vi "gxml_BlindXMLtoFlatString.vi"(6 "Encaps Array Info":T1, 8 "error in":errorcluster, 9 "Item Name":cluster{"Hierarchy":string, "Item Name":string}, 10 "Datatype":string, 11 "Item Contents":string) -> (0 "error out":errorcluster, 2 "XML Data (Flat Str)":string)   [LabVIEW 2011, in "Third Party VIs.lvlib" / "GXML.lvlib"]
uses:
  GXML.lvlib
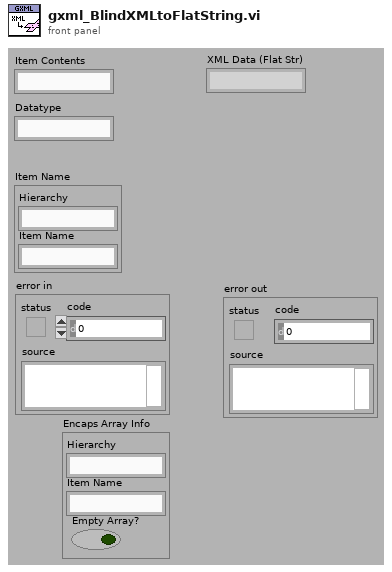
[diagram p1: front panel]
types:
  T1 = cluster{"Hierarchy":string, "Item Name":string, "Empty Array?":bool}
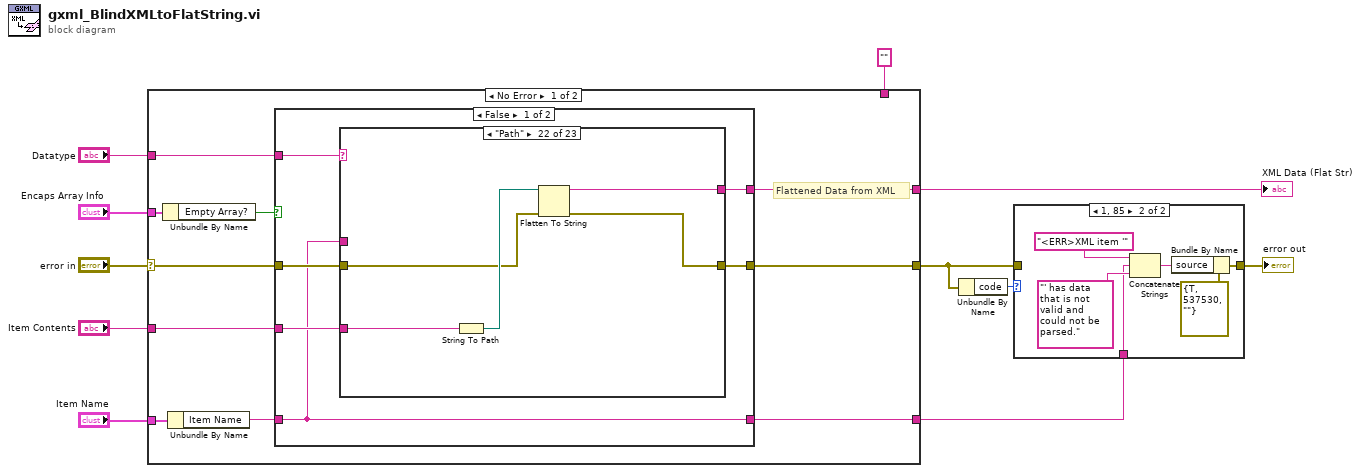
[diagram p0: block diagram]
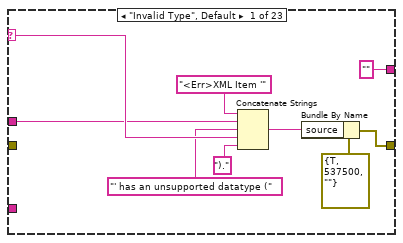
[diagram p3: hidden frame]
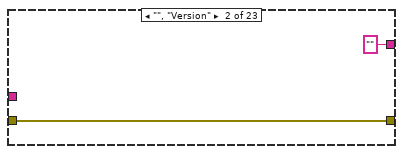
[diagram p4: hidden frame]
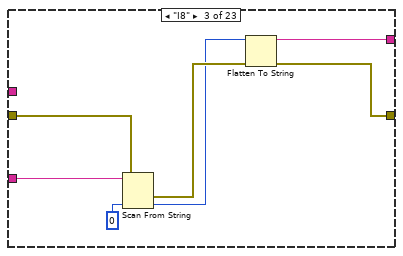
[diagram p5: hidden frame]
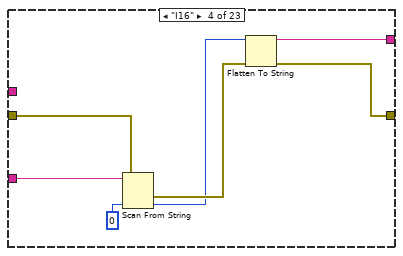
[diagram p6: hidden frame]
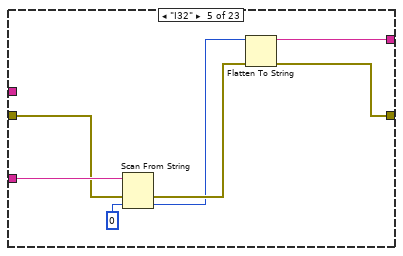
[diagram p7: hidden frame]
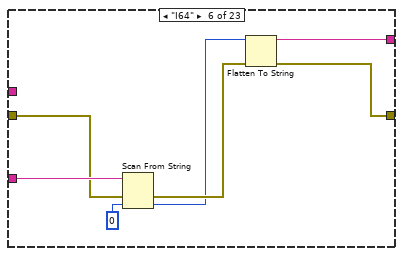
[diagram p8: hidden frame]
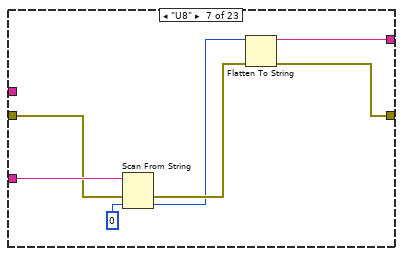
[diagram p9: hidden frame]
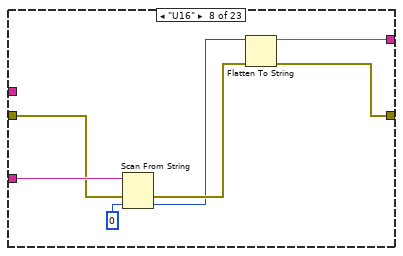
[diagram p10: hidden frame]
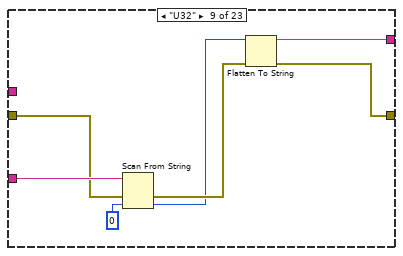
[diagram p11: hidden frame]
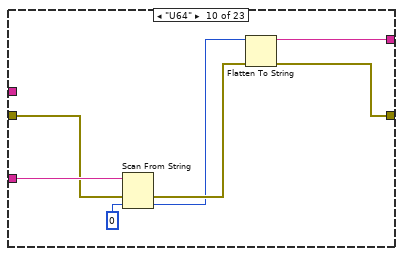
[diagram p12: hidden frame]
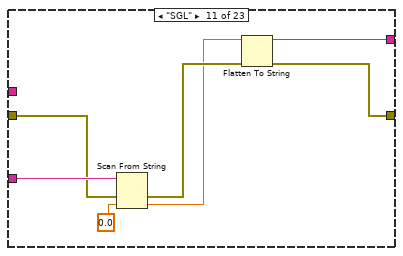
[diagram p13: hidden frame]
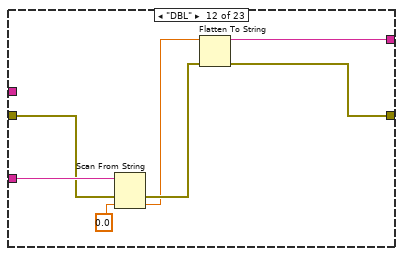
[diagram p14: hidden frame]
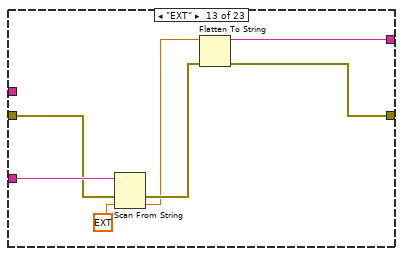
[diagram p15: hidden frame]
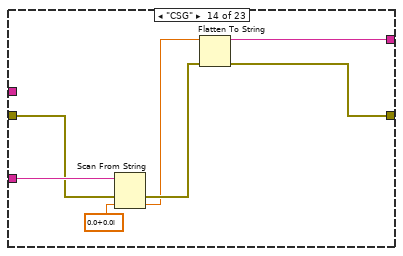
[diagram p16: hidden frame]
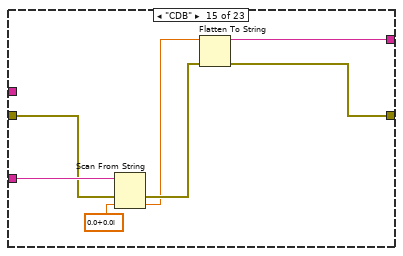
[diagram p17: hidden frame]
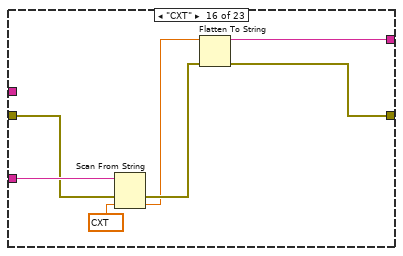
[diagram p18: hidden frame]
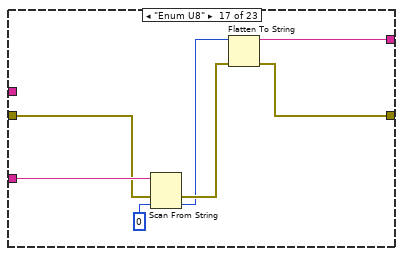
[diagram p19: hidden frame]
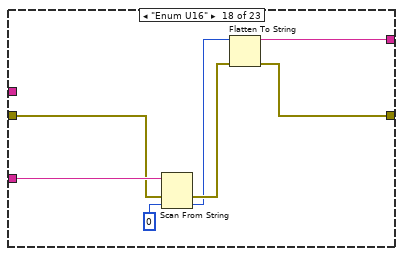
[diagram p20: hidden frame]
diagram:
  n1 = case shown="No Error" "error in" {
    selector: "error in" -> [w17 w191]
    tunnel: [w20 w191] -> w5
    tunnel: [w21 w190] -> w11
    tunnel: "Datatype" -> [w18 _]
    tunnel: "Item Contents" -> [w19 _]
    tunnel: "" ("data string") -> [_ w190]
    tunnel: "Item Name" -> [w16 _]
    tunnel: [w13 w190] -> w2
    tunnel: "Encaps Array Info" -> [w14 _]
    frame No Error {
      # "Flattened Data from XML"
      n2 = Unbundle By Name(w14) -> ("Empty Array?"=w12:bool)
      n3 = Unbundle By Name(w16) -> ("Item Name"=w15:string)
      n4 = case shown="False" w12 {
        tunnel: [w27 "" ("data string")] -> w21
        tunnel: [w26 w188] -> w20
        tunnel: w19 -> [w25 _]
        tunnel: w18 -> [w24 _]
        tunnel: w17 -> [w23 w188]
        tunnel: w15 -> [w22 w189]
        tunnel: [w22 w189] -> w13
        frame False {
          n5 = case shown="\"Path\"" w24 {
            selector: w24 -> [w33 _ _ _ _ _ _ _ _ _ _ _ _ _ _ _ _ _ _ _ _ _ _]
            tunnel: ["" ("data string") "" ("data string") w42 w49 w56 w63 w70 w77 w84 w91 w100 w107 w114 w121 w128 w135 w140 w147 w154 w163 w168 w173 w185] -> w27
            tunnel: [w34 w38 w41 w48 w55 w62 w69 w76 w83 w90 w101 w108 w115 w122 w129 w136 w137 w144 w152 w164 w169 w174 w186] -> w26
            tunnel: w25 -> [_ _ w44 w51 w58 w65 w72 w79 w86 w93 w98 w105 w112 w119 w126 w133 w143 w150 w157 w162 w165 w172 w178]
            tunnel: w23 -> [_ w38 w43 w50 w57 w64 w71 w78 w85 w92 w95 w102 w109 w116 w123 w130 w138 w145 w151 w158 w167 w170 w179]
            tunnel: w22 -> [w28 _ _ _ _ _ _ _ _ _ _ _ _ _ _ _ _ _ _ _ _ _ w177]
            frame "Invalid Type", Default {
              n6 = Concatenate Strings("<Err>XML Item '", w28, "' has an unsupported datatype (" ("string"), w33, ")." ("string")) -> (w32:string)
              n7 = Bundle By Name(cluster=errorcluster {"status"=TRUE, "code"=537500, "source"=""} ("error out"), "source"=w32) -> (w34:errorcluster)
            }
            frame "", "Version" {
            }
            frame "I8" {
              n8 = Scan From String(input string=w44, error in=w43, default 1=i8 0) -> (error out=w40:errorcluster, output 1=w39:i8)  [unwired: 2 in, 2 out]
              n9 = Flatten To String(anything=w39, error in (no error)=w40) -> (data string=w42:string, error out=w41:errorcluster)  [unwired: 2 in, 1 out]
            }
            frame "I16" {
              n10 = Scan From String(input string=w51, error in=w50, default 1=i16 0) -> (error out=w47:errorcluster, output 1=w46:i16)  [unwired: 2 in, 2 out]
              n11 = Flatten To String(anything=w46, error in (no error)=w47) -> (data string=w49:string, error out=w48:errorcluster)  [unwired: 2 in, 1 out]
            }
            frame "I32" {
              n12 = Scan From String(input string=w58, error in=w57, default 1=0) -> (error out=w54:errorcluster, output 1=w53:i32)  [unwired: 2 in, 2 out]
              n13 = Flatten To String(anything=w53, error in (no error)=w54) -> (data string=w56:string, error out=w55:errorcluster)  [unwired: 2 in, 1 out]
            }
            frame "I64" {
              n14 = Scan From String(input string=w65, error in=w64, default 1=i64 0) -> (error out=w61:errorcluster, output 1=w60:i64)  [unwired: 2 in, 2 out]
              n15 = Flatten To String(anything=w60, error in (no error)=w61) -> (data string=w63:string, error out=w62:errorcluster)  [unwired: 2 in, 1 out]
            }
            frame "U8" {
              n16 = Scan From String(input string=w72, error in=w71, default 1=u8 0) -> (error out=w68:errorcluster, output 1=w67:u8)  [unwired: 2 in, 2 out]
              n17 = Flatten To String(anything=w67, error in (no error)=w68) -> (data string=w70:string, error out=w69:errorcluster)  [unwired: 2 in, 1 out]
            }
            frame "U16" {
              n18 = Scan From String(input string=w79, error in=w78, default 1=u16 0) -> (error out=w75:errorcluster, output 1=w74:u16)  [unwired: 2 in, 2 out]
              n19 = Flatten To String(anything=w74, error in (no error)=w75) -> (data string=w77:string, error out=w76:errorcluster)  [unwired: 2 in, 1 out]
            }
            frame "U32" {
              n20 = Scan From String(input string=w86, error in=w85, default 1=u32 0) -> (error out=w82:errorcluster, output 1=w81:u32)  [unwired: 2 in, 2 out]
              n21 = Flatten To String(anything=w81, error in (no error)=w82) -> (data string=w84:string, error out=w83:errorcluster)  [unwired: 2 in, 1 out]
            }
            frame "U64" {
              n22 = Scan From String(input string=w93, error in=w92, default 1=u64 0) -> (error out=w89:errorcluster, output 1=w88:u64)  [unwired: 2 in, 2 out]
              n23 = Flatten To String(anything=w88, error in (no error)=w89) -> (data string=w91:string, error out=w90:errorcluster)  [unwired: 2 in, 1 out]
            }
            frame "SGL" {
              n24 = Scan From String(input string=w98, error in=w95, default 1=sgl 0.0) -> (error out=w97:errorcluster, output 1=w96:sgl)  [unwired: 2 in, 2 out]
              n25 = Flatten To String(anything=w96, error in (no error)=w97) -> (data string=w100:string, error out=w101:errorcluster)  [unwired: 2 in, 1 out]
            }
            frame "DBL" {
              n26 = Scan From String(input string=w105, error in=w102, default 1=0.0) -> (error out=w104:errorcluster, output 1=w103:dbl)  [unwired: 2 in, 2 out]
              n27 = Flatten To String(anything=w103, error in (no error)=w104) -> (data string=w107:string, error out=w108:errorcluster)  [unwired: 2 in, 1 out]
            }
            frame "EXT" {
              n28 = Scan From String(input string=w112, error in=w109, default 1=ext 0.0) -> (error out=w111:errorcluster, output 1=w110:ext)  [unwired: 2 in, 2 out]
              n29 = Flatten To String(anything=w110, error in (no error)=w111) -> (data string=w114:string, error out=w115:errorcluster)  [unwired: 2 in, 1 out]
            }
            frame "CSG" {
              n30 = Scan From String(input string=w119, error in=w116, default 1=csg 0.0+0.0i) -> (error out=w118:errorcluster, output 1=w117:csg)  [unwired: 2 in, 2 out]
              n31 = Flatten To String(anything=w117, error in (no error)=w118) -> (data string=w121:string, error out=w122:errorcluster)  [unwired: 2 in, 1 out]
            }
            frame "CDB" {
              n32 = Scan From String(input string=w126, error in=w123, default 1=cdb 0.0+0.0i) -> (error out=w125:errorcluster, output 1=w124:cdb)  [unwired: 2 in, 2 out]
              n33 = Flatten To String(anything=w124, error in (no error)=w125) -> (data string=w128:string, error out=w129:errorcluster)  [unwired: 2 in, 1 out]
            }
            frame "CXT" {
              n34 = Scan From String(input string=w133, error in=w130, default 1=cxt 0.0+0.0i) -> (error out=w132:errorcluster, output 1=w131:cxt)  [unwired: 2 in, 2 out]
              n35 = Flatten To String(anything=w131, error in (no error)=w132) -> (data string=w135:string, error out=w136:errorcluster)  [unwired: 2 in, 1 out]
            }
            frame "Enum U8" {
              n36 = Scan From String(input string=w143, error in=w138, default 1=u8 0) -> (error out=w141:errorcluster, output 1=w139:u8)  [unwired: 2 in, 2 out]
              n37 = Flatten To String(anything=w139, error in (no error)=w141) -> (data string=w140:string, error out=w137:errorcluster)  [unwired: 2 in, 1 out]
            }
            frame "Enum U16" {
              n38 = Scan From String(input string=w150, error in=w145, default 1=u16 0) -> (error out=w148:errorcluster, output 1=w146:u16)  [unwired: 2 in, 2 out]
              n39 = Flatten To String(anything=w146, error in (no error)=w148) -> (data string=w147:string, error out=w144:errorcluster)  [unwired: 2 in, 1 out]
            }
            frame "Enum U32" {
              n40 = Scan From String(input string=w157, error in=w151, default 1=u32 0) -> (error out=w155:errorcluster, output 1=w153:u32)  [unwired: 2 in, 2 out]
              n41 = Flatten To String(anything=w153, error in (no error)=w155) -> (data string=w154:string, error out=w152:errorcluster)  [unwired: 2 in, 1 out]
            }
            frame "Bool" {
              n42 = Scan From String(input string=w162, error in=w158, default 1=FALSE) -> (error out=w160:errorcluster, output 1=w159:bool)  [unwired: 2 in, 2 out]
              n43 = Flatten To String(anything=w159, error in (no error)=w160) -> (data string=w163:string, error out=w164:errorcluster)  [unwired: 2 in, 1 out]
            }
            frame "String", "Tag" {
              n44 = call "gxml_UnescapeChar.vi"("XML In"=w165) -> ("XML Out"=w166:string)  [unwired: 10 in]
              n45 = Flatten To String(anything=w166, error in (no error)=w167) -> (data string=w168:string, error out=w169:errorcluster)  [unwired: 2 in, 1 out]
            }
            frame "Path" {
              n46 = String To Path(string=w172) -> (path=w171:path)
              n47 = Flatten To String(anything=w171, error in (no error)=w170) -> (data string=w173:string, error out=w174:errorcluster)  [unwired: 2 in, 1 out]
            }
            frame "Time" {
              w176 = "'" ("string")
              n48 = Concatenate Strings(w176, w177, w176) -> (w175:string)
              n49 = call "gxml_TimeCheck.vi"("error in"=w179, "Time String"=w178, "Item Name"=w175) -> ("error out"=w180:errorcluster)  [unwired: 7 in]
              n50 = Scan From String(format string="%<%H:%M:%S %x>T", input string=w178, error in=w180, default 1=timestamp(0 s since 1904-01-01) ("time stamp")) -> (error out=w182:errorcluster, output 1=w184:timestamp)  [unwired: 1 in, 2 out]
              n51 = Flatten To String(anything=w184, error in (no error)=w182) -> (data string=w185:string, error out=w186:errorcluster)  [unwired: 2 in, 1 out]
            }
          }
        }
        frame True {
        }
      }
    }
    frame Error {
    }
  }
  "XML Data (Flat Str)" <- w11
  n52 = Unbundle By Name(w5) -> ("code"=w4:i32)
  n53 = case shown="1, 85" w4 {
    tunnel: w5 -> [w192 _]
    tunnel: [w192 w195] -> w6
    tunnel: w2 -> [_ w193]
    frame Default {
    }
    frame 1, 85 {
      n54 = Concatenate Strings("<ERR>XML item '" ("Format String"), w193, "' has data that is not valid and could not be parsed." ("Format String")) -> (w196:string)
      n55 = Bundle By Name(cluster=errorcluster {"status"=TRUE, "code"=537530, "source"=""} ("error in"), "source"=w196) -> (w195:errorcluster)
    }
  }
  "error out" <- w6
